vi "Create.vi"   [LabVIEW 2020, in "CSM-Helper.lvclass"]
uses:
  CSM-Helper.lvclass
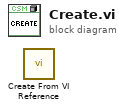
[diagram p0: block diagram]
diagram:
  n1 = call "Create From VI Reference.vi"() -> ()  [unwired: 10 in, 2 out]
